vi "Delete DVR.vi"(8 "Error In":errorcluster, 10 "Data Type DVR Refs":T1[](array[typedef]), 11 "Communication DVR Refs":T2[](array[typedef])) -> (0 "Error Out":errorcluster)   [LabVIEW 2023, in "Communication.lvclass"]
doc: "This method deletes the data value references of the communication class and calls another method to delete the DVrs of data class."
uses:
  Communication.lvclass
  Controls/Communication Class Details.ctl
  Controls/Data Class Details.ctl
  Data/Data.lvclass
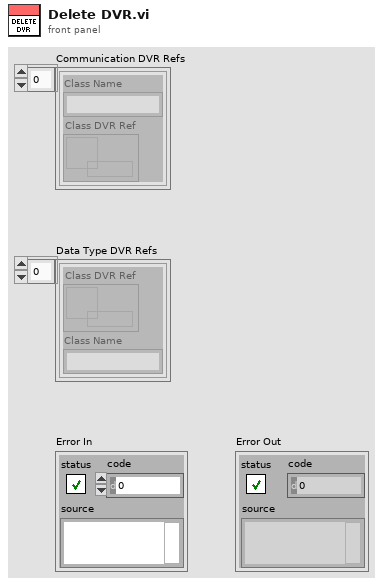
[diagram p1: front panel]
types:
  T1 = typedef "Data Class Details.ctl" = cluster{"Class DVR Ref":refnum<data-value>, "Class Name":string}
  T2 = typedef "Communication Class Details.ctl" = cluster{"Class Name":string, "Class DVR Ref":refnum<data-value>}
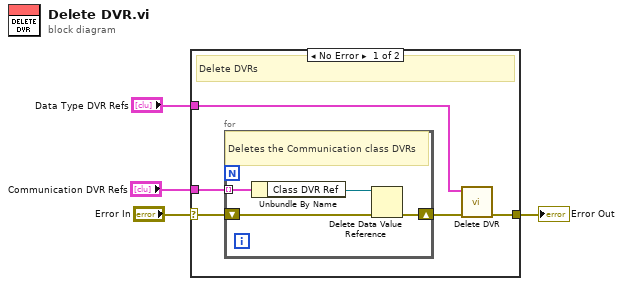
[diagram p0: block diagram]
diagram:
  n1 = case shown="No Error" "Error In" {
    selector: "Error In" -> [w9 w14]
    tunnel: [w6 w14] -> w3
    tunnel: "Communication DVR Refs" -> [w8 _]
    tunnel: "Data Type DVR Refs" -> [w5 _]
    frame No Error {
      # "Delete DVRs"
      n2 = for {
        shift-right: [w12] -> w7
        shift-left: w9 -> [w13]
        tunnel: w8 -> [w11] mode=indexing
        # "Deletes the Communication class DVRs"
        n3 = Unbundle By Name(w11) -> ("Class DVR Ref"=w10:refnum<data-value>)
        n4 = Delete Data Value Reference(data value reference=w10, error in=w13) -> (error out=w12:errorcluster)  [unwired: 1 out]
      }
      n5 = call "Delete DVR.vi"("Error In"=w7, "Data Type DVR Refs"=w5) -> ("Error Out"=w6:errorcluster)  [unwired: 9 in]
    }
    frame Error {
    }
  }
  "Error Out" <- w3
